vi "CentralStorage.Init.vi"(8 "error in (no error)":errorcluster, 10 "OwnQueue":refnum<queue>, 11 "CentralStorage in":refnum<data-value>) -> (0 "error out":errorcluster, 3 "CentralStorage out":refnum<data-value>)   [LabVIEW 2016, in "CentralStorage.lvclass"]
uses:
  CentralStorage.lvclass
  Package Libraries/Message Queue/private/MessageQueue.MessageTypeDef.ctl
  CentralStorage.lvclass/CentralStorage.ctl
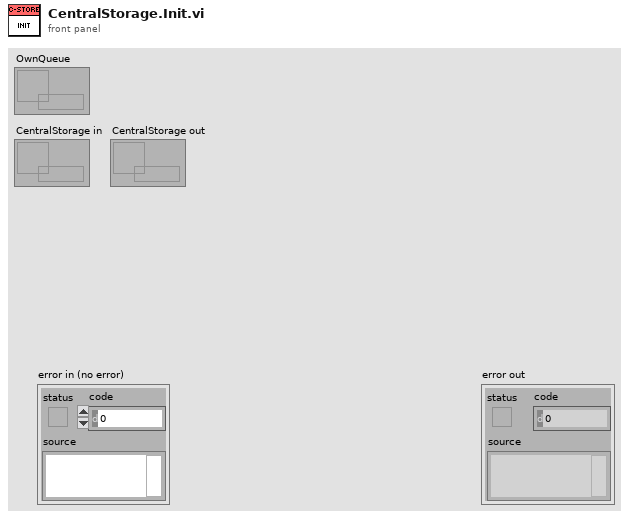
[diagram p1: front panel]
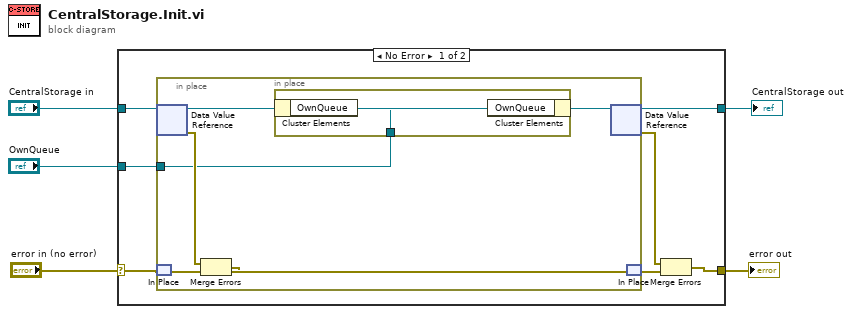
[diagram p0: block diagram]
diagram:
  n1 = case shown="No Error" "error in (no error)" {
    selector: "error in (no error)" -> [w9 w19]
    tunnel: [w8 w19] -> w5
    tunnel: [w10 w18] -> w2
    tunnel: "CentralStorage in" -> [w10 w18]
    tunnel: "OwnQueue" -> [w6 _]
    frame No Error {
      n2 = in-place {
        in-place-border: w6 -> [w12]
        n3 = in-place-dvr #1(w10) -> (w13:refnum<class "CentralStorage.lvclass">, w16:errorcluster)
        n4 = in-place-match #2(w9) -> (w15:errorcluster)
        n5 = Merge Errors(w16, w15) -> (w14:errorcluster)
        n6 = in-place {
          in-place-border: w12 -> [w17]
          n7 = in-place-cluster #3(w13) -> ()  [unwired: 1 out]
          n8 = in-place-cluster #3("OwnQueue"=w17) -> (w11:refnum<class "CentralStorage.lvclass">)
        }
        n9 = in-place-dvr #1(w11) -> (w7:errorcluster)  [unwired: 1 out]
        n10 = in-place-match #2(w14) -> ()  [unwired: 1 out]
      }
      n11 = Merge Errors(w7, w9) -> (w8:errorcluster)
    }
    frame Error {
    }
  }
  "error out" <- w5
  "CentralStorage out" <- w2
